vi "ReadHeader_Path.vi"(8 "datalog path (use dialog)":path) -> (0 "Offsets Array":T1, 2 "TTB Array (ms)\ntime axis (ms)\n0,1/fs,2/fs,...,n/fs":u32[](array[numeric]), 3 "Region height":i32, 4 "Header file data":T4 {"Pixel depth" items=["8 bits", "16 bits", "Float", "Complex", "RGB", "HSL"]; "time of 1st frame, \nsec since 1/1/04" format="%.2f"}, 5 "Region width":i32)   [LabVIEW 2014]
uses:
  4.Other/header ctl/Header file data.ctl
  4.Other/header ctl/Offset table.ctl
  4.Other/header ctl/Offset.ctl
  4.Other/header ctl/file number.ctl
panel:
  out "#frame":i32
  out "size(s)":i32
  out "file number":T3
  out "offset":T2
  out "Pixel depth":u32
  out "time of 1st frame, \nsec since 1/1/04":dbl
  out "Element 0 of TTB":u32
  out "Frames Acquired":u32
  in  "Header file data 2":T4 {"Pixel depth" items=["8 bits", "16 bits", "Float", "Complex", "RGB", "HSL"]; "time of 1st frame, \nsec since 1/1/04" format="%.2f"}
  # "Note : \n1. Glimpse bug \n frames acquired not match to file size\n2. frames acquired, size of TTB and size of offset array shoud be equal"
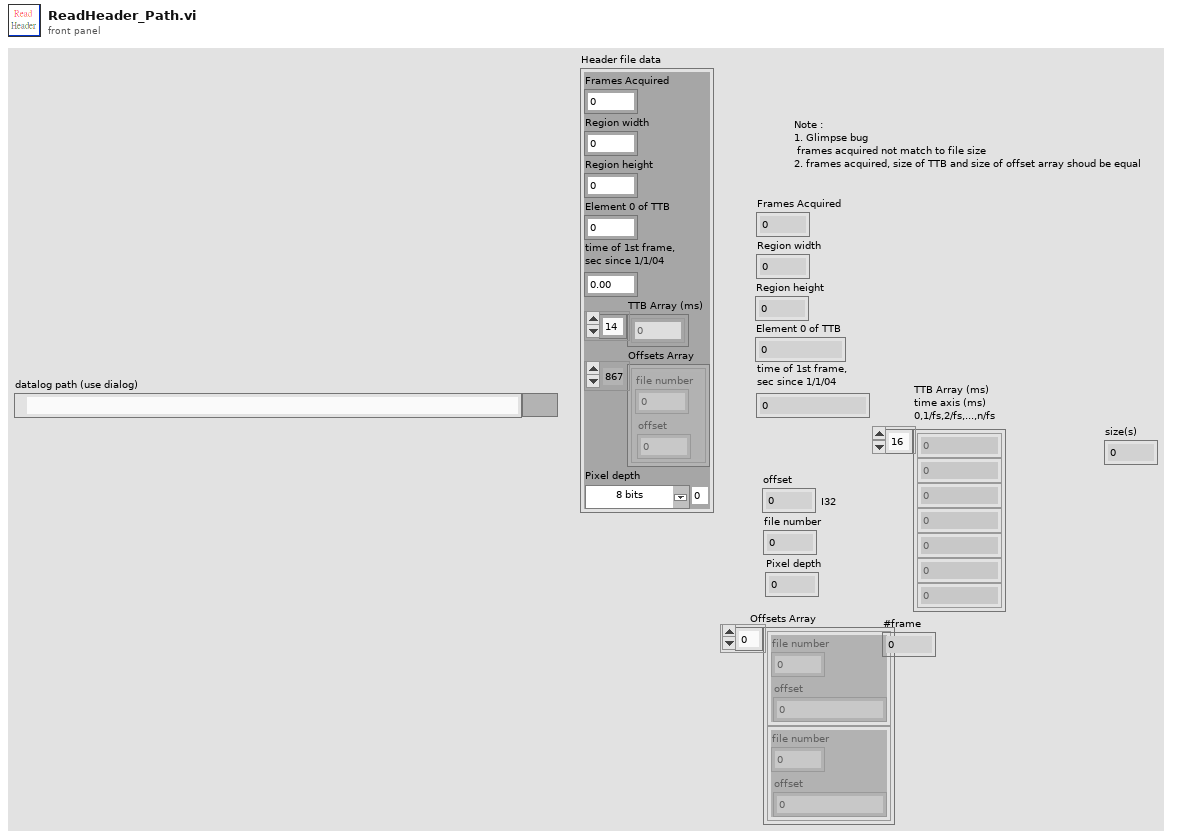
[diagram p1: front panel]
types:
  T1 = typedef "Offset table.ctl" = cluster{"offset":T2, "file number":T3}[]
  T2 = typedef "Offset.ctl" = i32
  T3 = typedef "file number.ctl" = u8
  T4 = typedef "Header file data.ctl" = cluster{"Frames Acquired":u32, "Region width":i32, "Region height":i32, "Element 0 of TTB":u32, "time of 1st frame, \nsec since 1/1/04":dbl, "TTB Array (ms)":u32[], "Offsets Array":T1, "Pixel depth":u32}
  T5 = enum16{"open", "replace", "create", "open or create", "replace or create", "replace or create with confirmation"}
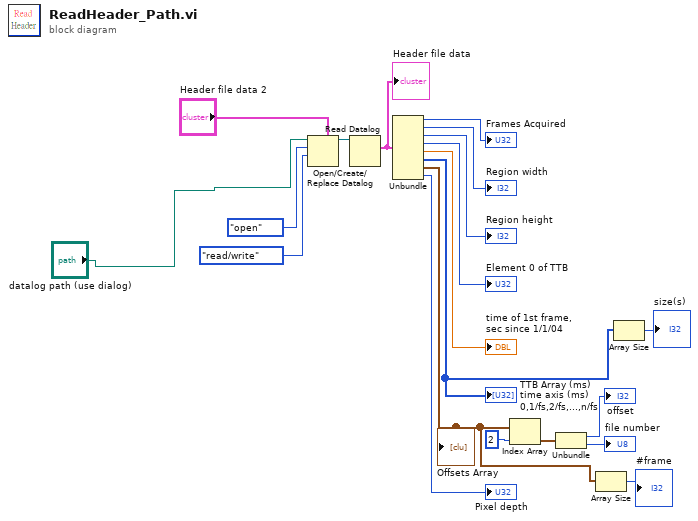
[diagram p0: block diagram]
diagram:
  n1 = Open/Create/Replace Datalog(5:"Header file data 2", 9:enum16{"read/write", "read-only", "write-only"}."read/write" ("access (0:read/write)"), 10:T5."open" ("operation (0:open)"), 11:"datalog path (use dialog)") -> (3:w18:refnum<k1>)  [unwired: 2 in, 2 out]
  n2 = Read Datalog(7:w18) -> (2:w16:T4)  [unwired: 2 in, 2 out]
  "Header file data" <- w16
  n3 = Unbundle(w16) -> ("Frames Acquired"=→"Frames Acquired":u32, "Region width"=→"Region width":i32, "Region height"=→"Region height":i32, "Element 0 of TTB"=→"Element 0 of TTB":u32, "time of 1st frame, \nsec since 1/1/04"=→"time of 1st frame, \nsec since 1/1/04":dbl, "TTB Array (ms)"=w5:u32[], "Offsets Array"=w2:T1, "Pixel depth"=→"Pixel depth":u32)
  "TTB Array (ms)\ntime axis (ms)\n0,1/fs,2/fs,...,n/fs" <- w5
  "Offsets Array" <- w2
  n4 = Index Array(array=w2, index=2) -> (element=w9:cluster{"offset":T2, "file number":T3})
  n5 = Unbundle(w9) -> ("offset"=→"offset":T2, "file number"=→"file number":T3)
  n6 = Array Size(array=w2) -> (size(s)=→"#frame":i32)
  n7 = Array Size(array=w5) -> (size(s)=→"size(s)":i32)
